vi "Handle.vi"(11 "jettl Queue Actor in":refnum<class "jettl Queue Actor.lvclass">) -> (2 "Destroy?":bool, 3 "jettl Queue Actor out":refnum<class "jettl Queue Actor.lvclass">)   [LabVIEW 2021, in "jettl.lvlib" / "jettl Queue Actor.lvclass"]
uses:
  jettl Queue Actor.lvclass
  C:/git/jettl/src/Actor/Queue Actor/Queue Actor.lvclass
  jettl Queue Actor.lvclass/jettl Queue Actor.ctl
  Queue State/Queue State/Queue State.lvclass
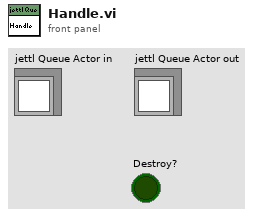
[diagram p1: front panel]
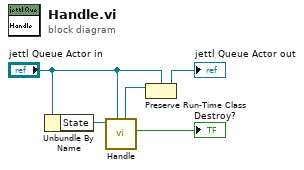
[diagram p0: block diagram]
diagram:
  n1 = Unbundle By Name("jettl Queue Actor in") -> ("State"=w5:refnum<class "Queue State.lvclass">)
  n2 = call-dynamic "Handle.vi"("Queue Actor in"="jettl Queue Actor in", "Queue State in"=w5) -> ("Destroy?"=→"Destroy?":bool, "Queue Actor out"=w4:refnum<class "Queue Actor.lvclass">)  [unwired: 8 in]
  n3 = Preserve Run-Time Class(object in=w4, 2:"jettl Queue Actor in") -> (object out=→"jettl Queue Actor out":refnum<class "jettl Queue Actor.lvclass">)  [unwired: 1 in, 1 out]
